vi "Reset.vi"(8 "error in (no error)":errorcluster, 11 "PWM in":refnum<class "LINX-PCA9865 PWM.lvclass">) -> (0 "error out":errorcluster, 3 "PWM out":refnum<class "LINX-PCA9865 PWM.lvclass">)   [LabVIEW 2019, in "LINX-PCA9865 PWM.lvclass"]
uses:
  LINX-PCA9865 PWM.lvclass
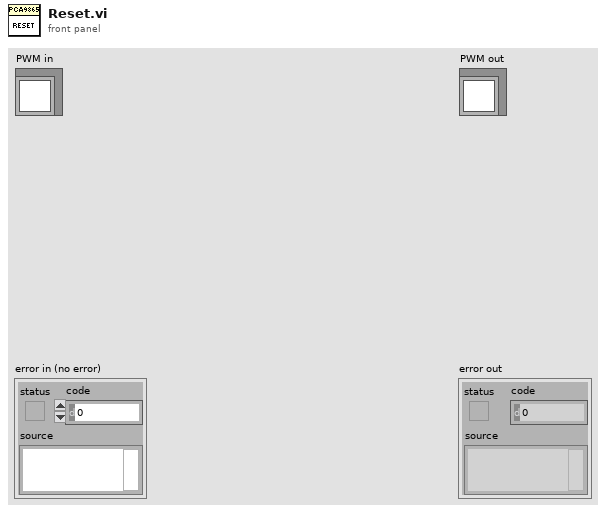
[diagram p1: front panel]
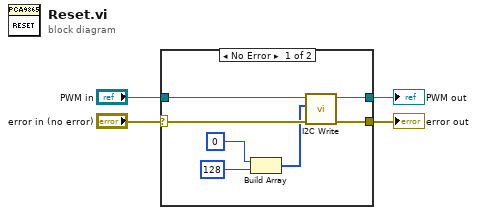
[diagram p0: block diagram]
diagram:
  n1 = case shown="No Error" "error in (no error)" {
    selector: "error in (no error)" -> [w10 w13]
    tunnel: [w6 w13] -> w3
    tunnel: [w7 w12] -> w1
    tunnel: "PWM in" -> [w11 w12]
    frame No Error {
      n2 = Build Array(u8 0 ("Address"), u8 128 ("Address")) -> (w9:u8[])
      n3 = call "I2C Write.vi"("error in (no error)"=w10, "Bytes to Write"=w9, "LINX-PCA9865 PWM in"=w11) -> ("error out"=w6:errorcluster, "LINX-PCA9865 PWM out"=w7:refnum<class "LINX-PCA9865 PWM.lvclass">)  [unwired: 7 in]
    }
    frame Error {
    }
  }
  "error out" <- w3
  "PWM out" <- w1
